vi "Initialise.vi"(8 "error in (no error)":errorcluster, 9 "Port":u16=502, 10 "IP Address":string="138.100.76.56", 11 "Robotiq in":refnum<class "Robotiq.lvclass">) -> (0 "error out":errorcluster, 3 "Robotiq out":refnum<class "Robotiq.lvclass">)   [LabVIEW 2013, in "Robotiq.lvclass"]
uses:
  Robotiq.lvclass
  Robotiq.lvclass/Robotiq.ctl
  <vilib>/NI Modbus.llb/MB Ethernet Master Query Write Single Register (poly).vi
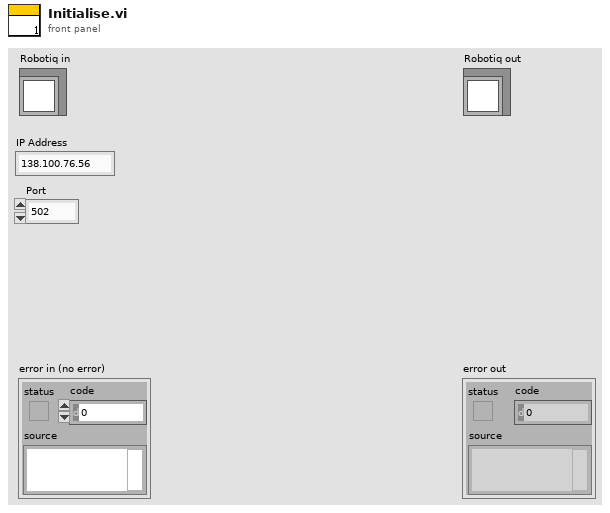
[diagram p1: front panel]
types:
  T1 = typedef "Gripper Status.ctl" = cluster{"Finger A":T2, "Finger B":T2, "Finger C":T2, "Scissor":T2, "Fault?":bool, "Activated?":bool}
  T2 = typedef "Finger Status.ctl" = cluster{"Position":dbl, "Current":dbl}
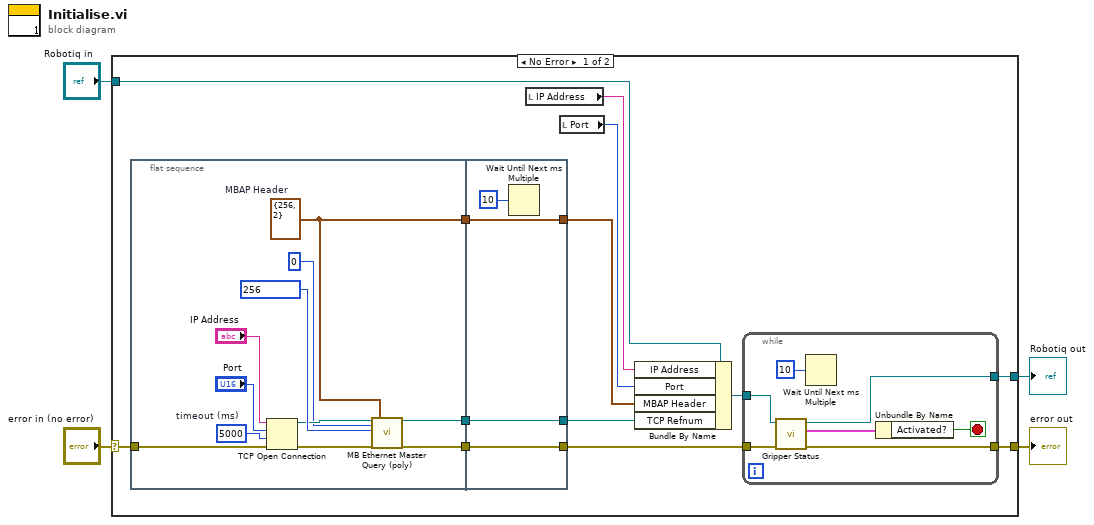
[diagram p0: block diagram]
diagram:
  n1 = case shown="No Error" "error in (no error)" {
    selector: "error in (no error)" -> [w14 w41]
    tunnel: [w5 w41] -> w3
    tunnel: [w7 w40] -> w1
    tunnel: "Robotiq in" -> [w13 w40]
    frame No Error {
      n2 = flat-sequence {
        tunnel: [w30] -> w17
        tunnel: [w29] -> w16
        tunnel: [w28] -> w15
        tunnel: w14 -> [w27]
        tunnel: [w38] -> w6
        tunnel: [w39] -> w9
        tunnel: w17 -> [w39]
        tunnel: w16 -> [w38]
        tunnel: [w36] -> w10
        tunnel: w15 -> [w36]
        frame #0 {
          w28 = cluster{"Transaction ID":u16, "Unit ID":u8} {"Transaction ID"=256, "Unit ID"=2}  # MBAP Header
          w34 = 5000  # timeout (ms)
          n3 = TCP Open Connection(address="IP Address", remote port or service name="Port", timeout ms (60000)=w34, error in (no error)=w27) -> (connection ID=w32:refnum<k5>, error out=w31:errorcluster)  [unwired: 1 in]
          n4 = call-poly <vilib>:"MB Ethernet Master Query (poly).vi"("TCP Connection Refnum in"=w32, "Address"=u16 0, "Register"=u16 256 ("Numeric"), "error in"=w31, "MBAP Header"=w28) -> ("TCP Connection Refnum (dup)"=w30:refnum<k5>, "error out"=w29:errorcluster)  [unwired: 12 in, 1 out]
        }
        frame #1 {
          n5 = Wait Until Next ms Multiple(millisecond multiple=u32 10) -> ()  [unwired: 1 out]
        }
      }
      n6 = local read "IP Address"() -> (w12:string)
      n7 = local read "Port"() -> (w11:u16)
      n8 = Bundle By Name(cluster=w13, "IP Address"=w12, "Port"=w11, "MBAP Header"=w10, "TCP Refnum"=w9) -> (w8:refnum<class "Robotiq.lvclass">)
      n9 = while {
        tunnel: w8 -> [w22]
        tunnel: [w21] -> w7
        tunnel: w6 -> [w20]
        tunnel: [w19] -> w5
        stop <- w23 stop-if-true
        n10 = call "Gripper Status.vi"("error in (no error)"=w20, "Robotiq in"=w22) -> ("error out"=w19:errorcluster, "Gripper Status"=w24:T1, "Robotiq out"=w21:refnum<class "Robotiq.lvclass">)  [unwired: 7 in]
        n11 = Wait Until Next ms Multiple(millisecond multiple=u32 10) -> ()  [unwired: 1 out]
        n12 = Unbundle By Name(w24) -> ("Activated?"=w23:bool)
      }
    }
    frame Error {
    }
  }
  "error out" <- w3
  "Robotiq out" <- w1
